vi "9606 Lower Bound not less than Upper Bound--error.vi"(8 "error in":errorcluster, 10 "Upper Bound":u16, 11 "Lower Bound":u16) -> (0 "error out":errorcluster)   [LabVIEW 2024, in "Electronic Datasheet.lvlib"]
uses:
  Electronic Datasheet.lvlib
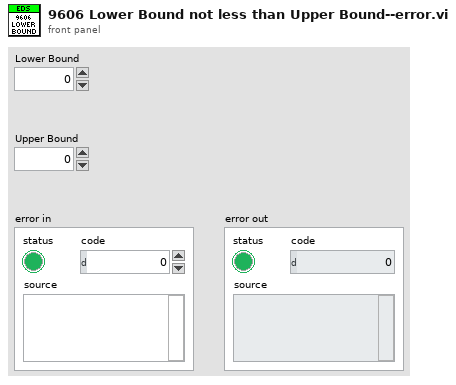
[diagram p1: front panel]
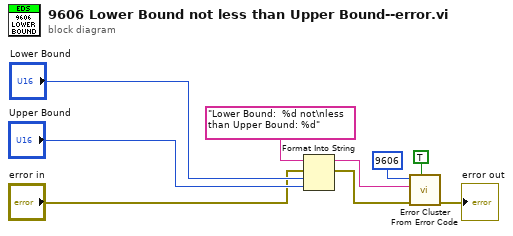
[diagram p0: block diagram]
diagram:
  n1 = Format Into String(initial string="Lower Bound:  %d not\nless than Upper Bound: %d" ("error message (\"\")"), error in="error in", "Lower Bound", "Upper Bound") -> (resulting string=w5:string, error out=w7:errorcluster)  [unwired: 1 in]
  n2 = call <vilib>:"Error Cluster From Error Code.vi"("show call chain? (False)"=TRUE, "error in (no error)"=w7, "error message (\"\")"=w5, "error code (0)"=9606) -> ("error out"=→"error out":errorcluster)  [unwired: 5 in]
